vi "set_Al_PID_01.vi"(0 "target flow (sccm)":dbl=76.0 format="%.2f", 1 "Run":bool, 2 "Bubbler In":bool, 3 "Active":bool=TRUE) -> ()   [LabVIEW 2011]
uses:
  <vilib>/Analysis/NI_AALPro.lvlib
panel:
  in  "dtDelay(s)":dbl=161845.394
  out "tTune(s)":dbl=161845.394
  out "Remote":bool
  out "prev dR":dbl
  out "dR":dbl
  out "Polynomial Coefficients":dbl[](array[numeric])=[-1.4185856873488687, 0.3207828308209371, 0.13144453708617976]
  out "Best Polynomial Fit":dbl[](array[numeric])=[-1.4185856873488687, -1.6139263817489564, -1.4535753275096295, -0.934721257482187, -0.06084472416107456, 1.168009538292087, 2.7539547788012695, 4.6979090060566655, 6.9965349595828625, 9.65378216839643, 12.656869913925354, 16.032582856357365, 19.766321537116767, 23.839791139200322, 28.29201256813708, 33.090057519195085, 38.231169600301214, 43.741895001434145, 49.604230522561835, 55.817258155180305, 63.621549699110574, 70.69684374251437, 78.07805746158404, 85.78401348130417, 93.89514333055536, 102.37353612475415, 111.1585051750553, 120.33168859799997, 129.86351160527155, 139.71949074374146, 149.9584374415381, 160.56464392932688, 171.50086747103902, 182.82343196442633, 194.50463604214053, 206.47125485701025, 218.94296295023602, 231.70008578092185, 244.74755627283324, 258.3136303817438]
  out "tFit_array":dbl[](array[numeric])=[-2.0, 0.0]
  out "RFit_array":dbl[](array[numeric])=[73.96843433835814, 74.61000000000001]
  out "error array":dbl[](array[numeric])=[-1.3899999999999864, -1.7800000000000011, -1.3500000000000085, -0.6200000000000045, 0.5699999999999932, 1.6099999999999994, 1.1999999999999886, 0.3199999999999932, -0.13000000000000966, -1.3700000000000045, -1.9499999999999886, -1.7399999999999949, -1.1200000000000045, -0.11999999999999034, 1.759999999999991, 2.3500000000000085, 2.1700000000000017, 1.4099999999999966, 0.4299999999999926, -0.6500000000000057, 54.959999999999994, 55.099999999999994, 55.66000000000001, 56.55000000000001, 57.02000000000001, 58.03, 58.129999999999995, 57.11999999999999, 56.599999999999994, 55.47, 54.80000000000001, 54.84, 55.129999999999995, 55.58, 57.16000000000001, 58.11, 58.09, 57.510000000000005, 56.74000000000001, 55.709999999999994]
  out "dt array":dbl[](array[numeric])=[0.0, -1.1669999999867287, -2.3260000000009313, -3.4940000000060536, -4.657999999995809, -5.820999999996275, -6.98499999998603, -8.14999999999418, -9.314000000013039, -10.478999999992084, -11.64000000001397, -12.807000000000698, -13.973999999987427, -15.135999999998603, -16.304000000003725, -17.469000000011874, -18.630999999993946, -19.796000000002095, -20.95999999999185, -22.122999999992317, -23.497999999992317, -24.67499999998836, -25.84299999999348, -27.005999999993946, -28.176000000006752, -29.347000000008848, -30.510999999998603, -31.679000000003725, -32.84700000000885, -34.0109999999986, -35.178000000014435, -36.345999999990454, -37.5109999999986, -38.679000000003725, -39.84700000000885, -41.00800000000163, -42.18299999998999, -43.35099999999511, -44.513000000006286, -45.68900000001304]
  out "Rtarget array":dbl[](array[numeric])=[76.0, 76.0, 76.0, 76.0, 76.0, 76.0, 76.0, 76.0, 76.0, 76.0, 76.0, 76.0, 76.0, 76.0, 76.0, 76.0, 76.0, 76.0, 76.0, 76.0, 20.0, 20.0, 20.0, 20.0, 20.0, 20.0, 20.0, 20.0, 20.0, 20.0, 20.0, 20.0, 20.0, 20.0, 20.0, 20.0, 20.0, 20.0, 20.0, 20.0]
  out "t array":dbl[](array[numeric])=[161845.394, 161844.227, 161843.068, 161841.9, 161840.736, 161839.573, 161838.409, 161837.244, 161836.08, 161834.915, 161833.754, 161832.587, 161831.42, 161830.258, 161829.09, 161827.925, 161826.763, 161825.598, 161824.434, 161823.271, 161821.896, 161820.719, 161819.551, 161818.388, 161817.218, 161816.047, 161814.883, 161813.715, 161812.547, 161811.383, 161810.216, 161809.048, 161807.883, 161806.715, 161805.547, 161804.386, 161803.211, 161802.043, 161800.881, 161799.705]
  out "R array":dbl[](array[numeric])=[74.61000000000001, 74.22, 74.64999999999999, 75.38, 76.57, 77.61, 77.19999999999999, 76.32, 75.86999999999999, 74.63, 74.05000000000001, 74.26, 74.88, 75.88000000000001, 77.75999999999999, 78.35000000000001, 78.17, 77.41, 76.42999999999999, 75.35, 74.96, 75.1, 75.66000000000001, 76.55000000000001, 77.02000000000001, 78.03, 78.13, 77.11999999999999, 76.6, 75.47, 74.80000000000001, 74.84, 75.13, 75.58, 77.16000000000001, 78.11, 78.09, 77.51, 76.74000000000001, 75.71]
  out "tuning":bool
  in  "Tune":bool
  in  "stop":bool
  in  "Ks":dbl
  out "dt(s)":dbl=1.1669999999867287
  out "windup error":dbl
  out "tPrev":dbl=161845.394
  out "target value":dbl=8.607079070006002
  out "error":dbl=-1.3899999999999864
  out "tNow(s)":dbl=161845.394
  out "weight array":dbl[](array[numeric])=[1.0, 0.3112994401423479, 0.09768570948263659, 0.03037911236430853, 0.009485414272106564, 0.0029646390229553033, 0.0009256632966347818, 0.00028873535962988374, 9.01532101455707e-05, 2.8120829299984297e-05, 8.806680295207305e-06, 2.741514645410681e-06, 8.534319742583924e-07, 2.6700458671159456e-07, 8.303530152421186e-08, 2.5900592293904588e-08, 8.103255033572197e-09, 2.5275888811806865e-09, 7.892010589399871e-10, 2.4666252724157755e-10, 6.236605368793774e-11, 1.9221339918994332e-11, 5.977611753902341e-12, 1.8682854076081917e-12, 5.79854027362869e-13, 1.7978764328562998e-13, 5.613594818436806e-14, 1.74576228867237e-14, 5.429116398891195e-15, 1.6951587510987664e-15, 5.277019701540894e-16, 1.6410913665416056e-16, 5.1189358768628024e-17, 1.5919291471855112e-17, 4.95071333304516e-18, 1.5504290109481995e-18, 4.788019052453027e-19, 1.4890178877471836e-19, 4.6585389077974155e-20, 1.437207306183795e-20]
  in  "# of points to watch":i32=60
  in  "tSmooth(s)":dbl=1.0
  out "first":bool
  out "XY Graph":cluster{"Value":dbl[], "Value":dbl[]}[](graph)=[{"Value"=[0.0, -1.1669999999867287, -2.3260000000009313, -3.4940000000060536, -4.657999999995809, -5.820999999996275, -6.98499999998603, -8.14999999999418, -9.314000000013039, -10.478999999992084, -11.64000000001397, -12.807000000000698, -13.973999999987427, -15.135999999998603, -16.304000000003725, -17.469000000011874, -18.630999999993946, -19.796000000002095, -20.95999999999185, -22.122999999992317, -23.497999999992317, -24.67499999998836, -25.84299999999348, -27.005999999993946, -28.176000000006752, -29.347000000008848, -30.510999999998603, -31.679000000003725, -32.84700000000885, -34.0109999999986, -35.178000000014435, -36.345999999990454, -37.5109999999986, -38.679000000003725, -39.84700000000885, -41.00800000000163, -42.18299999998999, -43.35099999999511, -44.513000000006286, -45.68900000001304], "Value"=[74.61000000000001, 74.22, 74.64999999999999, 75.38, 76.57, 77.61, 77.19999999999999, 76.32, 75.86999999999999, 74.63, 74.05000000000001, 74.26, 74.88, 75.88000000000001, 77.75999999999999, 78.35000000000001, 78.17, 77.41, 76.42999999999999, 75.35, 74.96, 75.1, 75.66000000000001, 76.55000000000001, 77.02000000000001, 78.03, 78.13, 77.11999999999999, 76.6, 75.47, 74.80000000000001, 74.84, 75.13, 75.58, 77.16000000000001, 78.11, 78.09, 77.51, 76.74000000000001, 75.71]}, {"Value"=[-2.0, 0.0], "Value"=[73.96843433835814, 74.61000000000001]}, {"Value"=[0.0, -1.1669999999867287, -2.3260000000009313, -3.4940000000060536, -4.657999999995809, -5.820999999996275, -6.98499999998603, -8.14999999999418, -9.314000000013039, -10.478999999992084, -11.64000000001397, -12.807000000000698, -13.973999999987427, -15.135999999998603, -16.304000000003725, -17.469000000011874, -18.630999999993946, -19.796000000002095, -20.95999999999185, -22.122999999992317, -23.497999999992317, -24.67499999998836, -25.84299999999348, -27.005999999993946, -28.176000000006752, -29.347000000008848, -30.510999999998603, -31.679000000003725, -32.84700000000885, -34.0109999999986, -35.178000000014435, -36.345999999990454, -37.5109999999986, -38.679000000003725, -39.84700000000885, -41.00800000000163, -42.18299999998999, -43.35099999999511, -44.513000000006286, -45.68900000001304], "Value"=[76.0, 76.0, 76.0, 76.0, 76.0, 76.0, 76.0, 76.0, 76.0, 76.0, 76.0, 76.0, 76.0, 76.0, 76.0, 76.0, 76.0, 76.0, 76.0, 76.0, 20.0, 20.0, 20.0, 20.0, 20.0, 20.0, 20.0, 20.0, 20.0, 20.0, 20.0, 20.0, 20.0, 20.0, 20.0, 20.0, 20.0, 20.0, 20.0, 20.0]}]
  out "current value":dbl=8.607079070006002
  in  "Period (s)":dbl=0.5
  out "dValue":dbl=2.1714937580001004
  out "derivative":dbl=0.3207828308209371
  out "integral":dbl=21701.037580001004
  in  "Kd":dbl
  in  "Ki":dbl=0.0001
  in  "Kp":dbl=0.001
  out "actual flow (sccm)":dbl=74.61000000000001 format="%.2f"
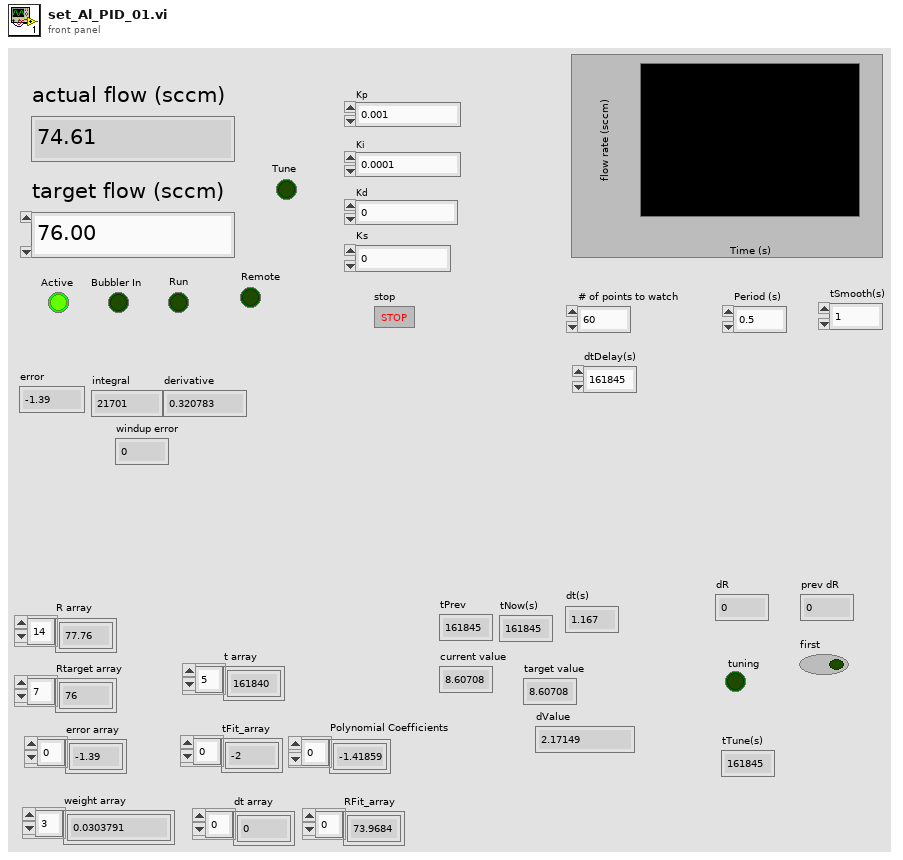
[diagram p1: front panel]
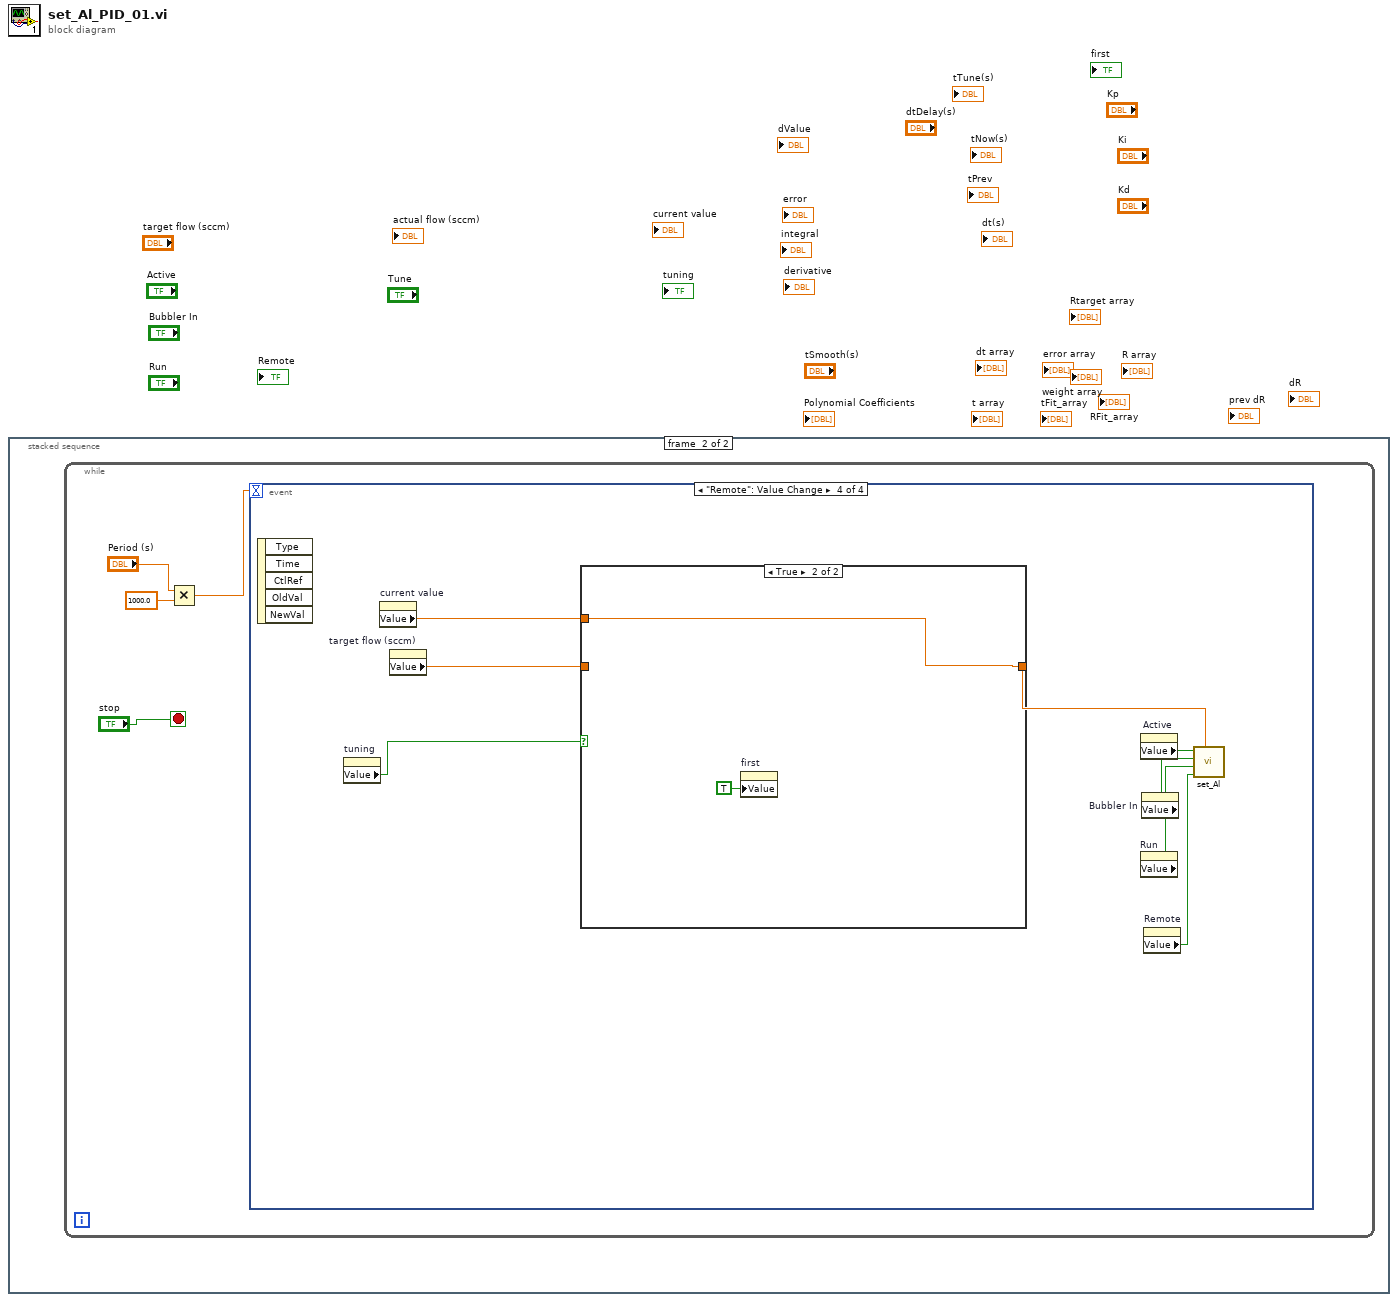
[diagram p0: block diagram]
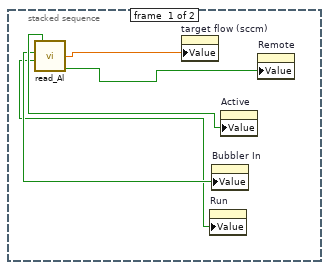
[diagram p2: hidden frame]
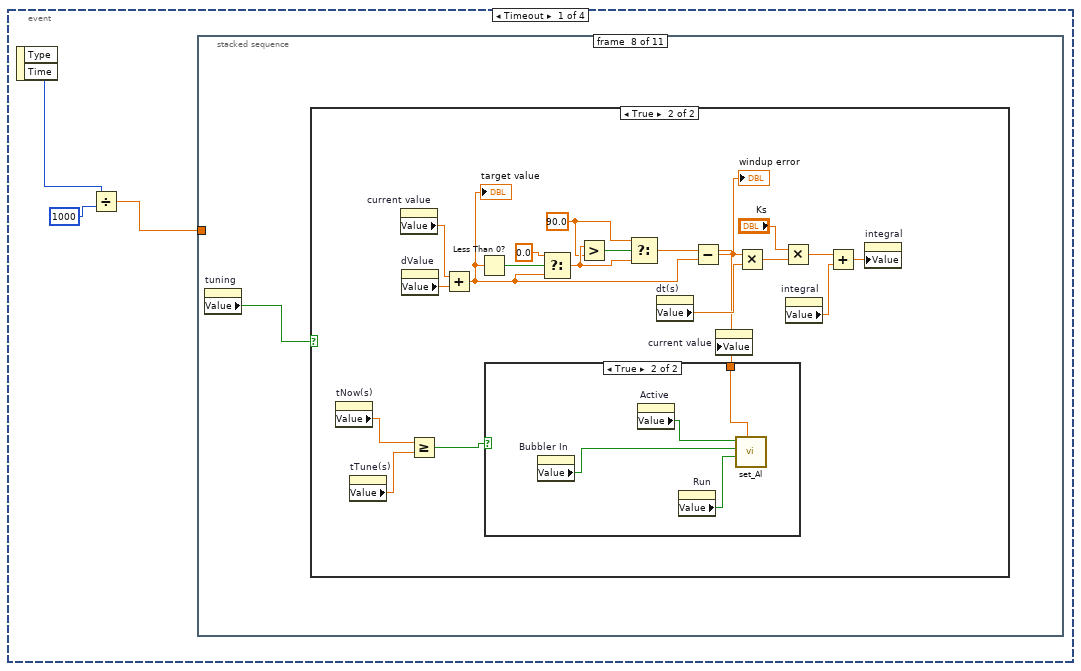
[diagram p3: hidden frame]
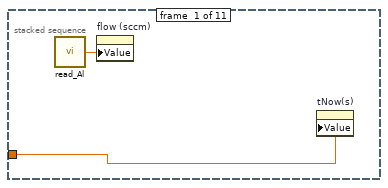
[diagram p4: hidden frame]
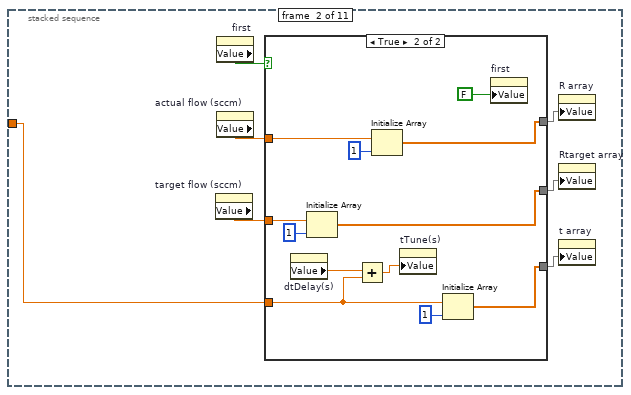
[diagram p5: hidden frame]
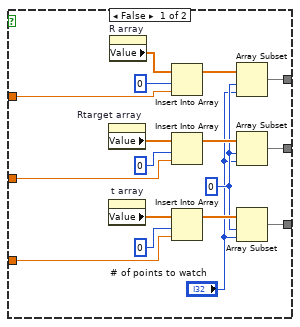
[diagram p6: hidden frame]
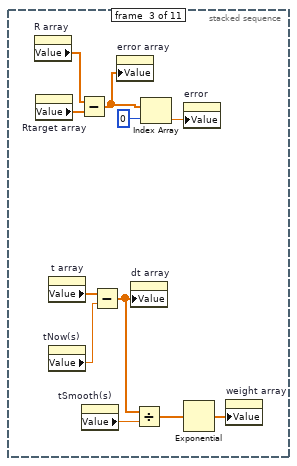
[diagram p7: hidden frame]
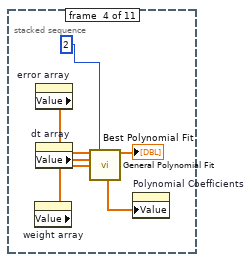
[diagram p8: hidden frame]
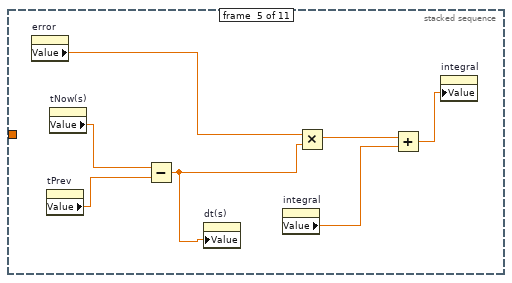
[diagram p9: hidden frame]
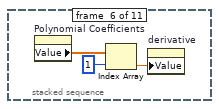
[diagram p10: hidden frame]
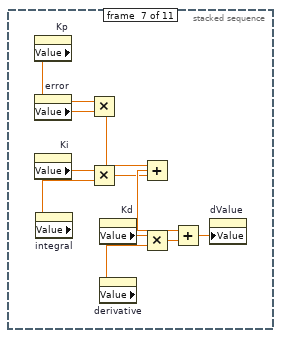
[diagram p11: hidden frame]
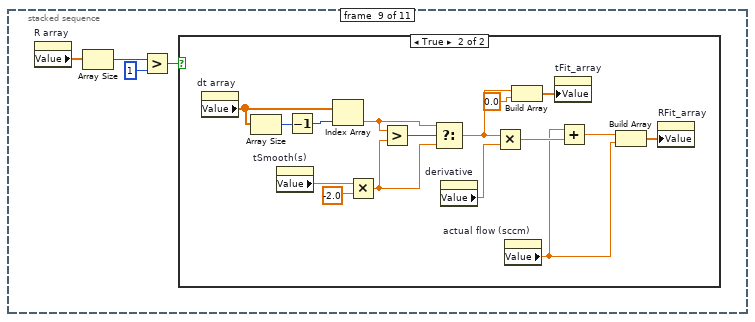
[diagram p14: hidden frame]
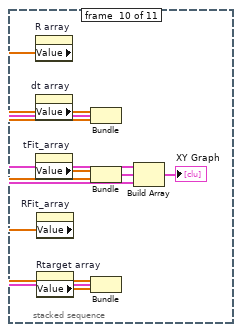
[diagram p16: hidden frame]
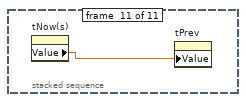
[diagram p17: hidden frame]
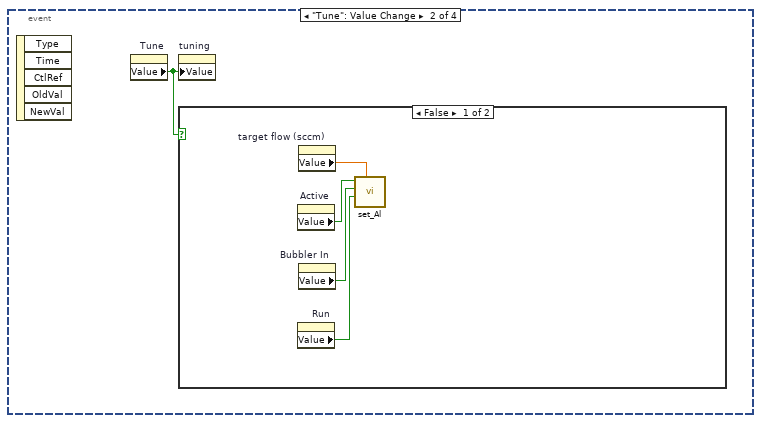
[diagram p18: hidden frame]
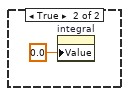
[diagram p19: hidden frame]
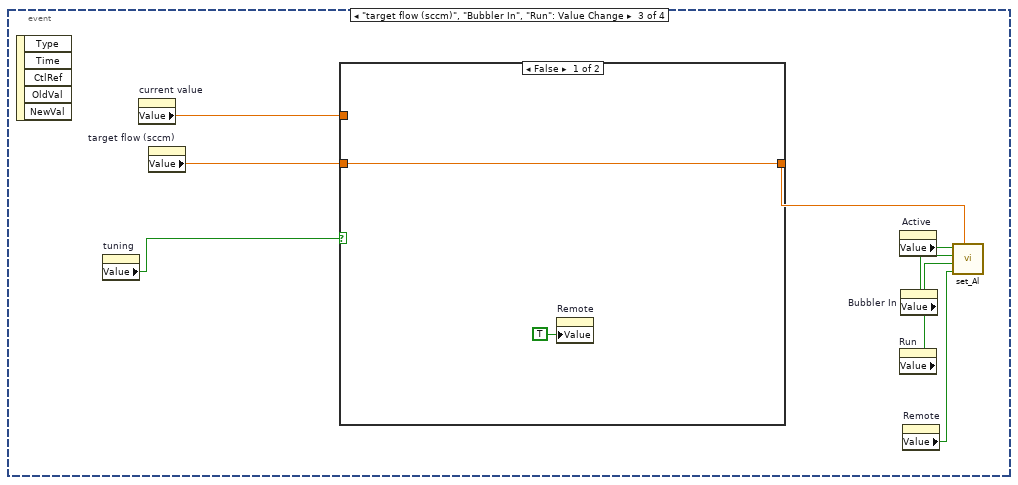
[diagram p20: hidden frame]
diagram:
  n1 = stacked-sequence {
    frame #0 {
      n2 = call "read_Al.vi"() -> ("ALMFC1"=w5:dbl, "Remote"=w1:bool, "Run"=w2:bool, "Bubbler In"=w3:bool, "Active"=w4:bool)
      n3 = property on="target flow (sccm)" class="DigNum (strict)"("Value"=w5) -> ()  [unwired: 2 in, 2 out]
      n4 = property on="Run" class="Bool (strict)"("Value"=w2) -> ()  [unwired: 2 in, 2 out]
      n5 = property on="Bubbler In" class="Bool (strict)"("Value"=w3) -> ()  [unwired: 2 in, 2 out]
      n6 = property on="Active" class="Bool (strict)"("Value"=w4) -> ()  [unwired: 2 in, 2 out]
      n7 = property on="Remote" class="Bool (strict)"("Value"=w1) -> ()  [unwired: 2 in, 2 out]
    }
    frame #1 {
      n8 = while {
        stop <- "stop" stop-if-true
        n9 = Multiply(x="Period (s)", y=1000.0) -> (x*y=w7:dbl)
        n10 = event shown="[3] \"Remote\": Value Change" {
          selector: _ -> [_ _ _ _]
          dyn-events: _ -> [_ _ _ _]
          timeout: w7 -> [_ _ _ _]
          event Timeout {
            n11 = event-data() -> ("Time"=w12:u32)  [unwired: 1 in, 1 out]
            n12 = Divide(x=w12, y=u32 1000) -> (x/y=w10:dbl)
            n13 = stacked-sequence {
              tunnel: w10 -> [w14 w21 _ _ _ _ _ _ _ _ _]
              frame #0 {
                n14 = call "read_Al.vi"() -> ("ALMFC1"=w13:dbl)  [unwired: 4 out]
                n15 = property on="flow (sccm)" class="DigNum (strict)"("Value"=w13) -> ()  [unwired: 2 in, 2 out]
                n16 = property on="tNow(s)" class="DigNum (strict)"("Value"=w14) -> ()  [unwired: 2 in, 2 out]
              }
              frame #1 {
                n17 = property on="target flow (sccm)" class="DigNum (strict)"() -> ("Value"=w16:dbl)  [unwired: 2 in, 2 out]
                n18 = property on="first" class="Bool (strict)"() -> ("Value"=w20:bool)  [unwired: 2 in, 2 out]
                n19 = property on="actual flow (sccm)" class="DigNum (strict)"() -> ("Value"=w19:dbl)  [unwired: 2 in, 2 out]
                n20 = case shown="True" w20 {
                  tunnel: w19 -> [w37 w49]
                  tunnel: [w28 w47] -> w18
                  tunnel: w21 -> [w34 w39]
                  tunnel: [w26 w45] -> w17
                  tunnel: w16 -> [w30 w43]
                  tunnel: [w24 w42] -> w15
                  frame False {
                    w23 = 0 ("index")
                    n21 = property on="Rtarget array" class="Arr (strict)"() -> ("Value"=w31:dbl[])  [unwired: 2 in, 2 out]
                    n22 = property on="t array" class="Arr (strict)"() -> ("Value"=w33:dbl[])  [unwired: 2 in, 2 out]
                    n23 = property on="R array" class="Arr (strict)"() -> ("Value"=w36:dbl[])  [unwired: 2 in, 2 out]
                    n24 = Insert Into Array(array=w36, index=0, new element=w37) -> (w29:dbl[])
                    n25 = Insert Into Array(array=w31, index=0, new element=w30) -> (w25:dbl[])
                    n26 = Insert Into Array(array=w33, index=0, new element=w34) -> (w27:dbl[])
                    n27 = Array Subset(array=w29, index=w23, length="# of points to watch") -> (w28:dbl[])
                    n28 = Array Subset(array=w25, index=w23, length="# of points to watch") -> (w24:dbl[])
                    n29 = Array Subset(array=w27, index=w23, length="# of points to watch") -> (w26:dbl[])
                  }
                  frame True {
                    n30 = property on="dtDelay(s)" class="DigNum (strict)"() -> ("Value"=w40:dbl)  [unwired: 2 in, 2 out]
                    n31 = Initialize Array(w43, 1 ("dimension size")) -> (w42:dbl[])
                    n32 = Add(x=w40, y=w39) -> (x+y=w41:dbl)
                    n33 = Initialize Array(w49, 1 ("dimension size")) -> (w47:dbl[])
                    n34 = property on="tTune(s)" class="DigNum (strict)"("Value"=w41) -> ()  [unwired: 2 in, 2 out]
                    n35 = Initialize Array(w39, 1 ("dimension size")) -> (w45:dbl[])
                    n36 = property on="first" class="Bool (strict)"("Value"=FALSE ("first")) -> ()  [unwired: 2 in, 2 out]
                  }
                }
                n37 = property on="R array" class="Arr (strict)"("Value"=w18) -> ()  [unwired: 2 in, 2 out]
                n38 = property on="Rtarget array" class="Arr (strict)"("Value"=w15) -> ()  [unwired: 2 in, 2 out]
                n39 = property on="t array" class="Arr (strict)"("Value"=w17) -> ()  [unwired: 2 in, 2 out]
              }
              frame #2 {
                n40 = property on="R array" class="Arr (strict)"() -> ("Value"=w55:dbl[])  [unwired: 2 in, 2 out]
                n41 = property on="Rtarget array" class="Arr (strict)"() -> ("Value"=w54:dbl[])  [unwired: 2 in, 2 out]
                n42 = property on="t array" class="Arr (strict)"() -> ("Value"=w61:dbl[])  [unwired: 2 in, 2 out]
                n43 = property on="tNow(s)" class="DigNum (strict)"() -> ("Value"=w60:dbl)  [unwired: 2 in, 2 out]
                n44 = Subtract(x=w55, y=w54) -> (x-y=w53:dbl[])
                n45 = property on="tSmooth(s)" class="DigNum (strict)"() -> ("Value"=w59:dbl)  [unwired: 2 in, 2 out]
                n46 = Subtract(x=w61, y=w60) -> (x-y=w57:dbl[])
                n47 = property on="error array" class="Arr (strict)"("Value"=w53) -> ()  [unwired: 2 in, 2 out]
                n48 = property on="dt array" class="Arr (strict)"("Value"=w57) -> ()  [unwired: 2 in, 2 out]
                n49 = Divide(x=w57, y=w59) -> (x/y=w58:dbl[])
                n50 = Index Array(array=w53, index=0) -> (element=w51:dbl)
                n51 = property on="error" class="DigNum (strict)"("Value"=w51) -> ()  [unwired: 2 in, 2 out]
                n52 = Exponential(1:w58) -> (0:w56:dbl[])
                n53 = property on="weight array" class="Arr (strict)"("Value"=w56) -> ()  [unwired: 2 in, 2 out]
              }
              frame #3 {
                n54 = property on="weight array" class="Arr (strict)"() -> ("Value"=w65:dbl[])  [unwired: 2 in, 2 out]
                n55 = property on="error array" class="Arr (strict)"() -> ("Value"=w67:dbl[])  [unwired: 2 in, 2 out]
                n56 = property on="dt array" class="Arr (strict)"() -> ("Value"=w66:dbl[])  [unwired: 2 in, 2 out]
                n57 = call <vilib>:"General Polynomial Fit.vi"("Y"=w67, "polynomial order"=2, "X"=w66, "Weight"=w65) -> ("Best Polynomial Fit"=→"Best Polynomial Fit":dbl[], "Polynomial Coefficients"=w62:dbl[])  [unwired: 8 in, 2 out]
                n58 = property on="Polynomial Coefficients" class="Arr (strict)"("Value"=w62) -> ()  [unwired: 2 in, 2 out]
              }
              frame #4 {
                n59 = property on="error" class="DigNum (strict)"() -> ("Value"=w70:dbl)  [unwired: 2 in, 2 out]
                n60 = property on="tPrev" class="DigNum (strict)"() -> ("Value"=w69:dbl)  [unwired: 2 in, 2 out]
                n61 = property on="tNow(s)" class="DigNum (strict)"() -> ("Value"=w68:dbl)  [unwired: 2 in, 2 out]
                n62 = Subtract(x=w68, y=w69) -> (x-y=w74:dbl)
                n63 = property on="dt(s)" class="DigNum (strict)"("Value"=w74) -> ()  [unwired: 2 in, 2 out]
                n64 = property on="integral" class="DigNum (strict)"() -> ("Value"=w72:dbl)  [unwired: 2 in, 2 out]
                n65 = Multiply(x=w70, y=w74) -> (x*y=w71:dbl)
                n66 = Add(x=w71, y=w72) -> (x+y=w73:dbl)
                n67 = property on="integral" class="DigNum (strict)"("Value"=w73) -> ()  [unwired: 2 in, 2 out]
              }
              frame #5 {
                n68 = property on="Polynomial Coefficients" class="Arr (strict)"() -> ("Value"=w77:dbl[])  [unwired: 2 in, 2 out]
                n69 = Index Array(array=w77, index=1) -> (element=w75:dbl)
                n70 = property on="derivative" class="DigNum (strict)"("Value"=w75) -> ()  [unwired: 2 in, 2 out]
              }
              frame #6 {
                n71 = property on="Kp" class="DigNum (strict)"() -> ("Value"=w78:dbl)  [unwired: 2 in, 2 out]
                n72 = property on="error" class="DigNum (strict)"() -> ("Value"=w88:dbl)  [unwired: 2 in, 2 out]
                n73 = property on="Ki" class="DigNum (strict)"() -> ("Value"=w79:dbl)  [unwired: 2 in, 2 out]
                n74 = property on="integral" class="DigNum (strict)"() -> ("Value"=w80:dbl)  [unwired: 2 in, 2 out]
                n75 = Multiply(x=w78, y=w88) -> (x*y=w83:dbl)
                n76 = Multiply(x=w79, y=w80) -> (x*y=w84:dbl)
                n77 = property on="Kd" class="DigNum (strict)"() -> ("Value"=w81:dbl)  [unwired: 2 in, 2 out]
                n78 = property on="derivative" class="DigNum (strict)"() -> ("Value"=w82:dbl)  [unwired: 2 in, 2 out]
                n79 = Add(x=w83, y=w84) -> (x+y=w86:dbl)
                n80 = Multiply(x=w81, y=w82) -> (x*y=w85:dbl)
                n81 = Add(x=w86, y=w85) -> (x+y=w87:dbl)
                n82 = property on="dValue" class="DigNum (strict)"("Value"=w87) -> ()  [unwired: 2 in, 2 out]
              }
              frame #7 {
                n83 = property on="tuning" class="Bool (strict)"() -> ("Value"=w89:bool)  [unwired: 2 in, 2 out]
                n84 = case shown="True" w89 {
                  frame False {
                  }
                  frame True {
                    w102 = 90.0 ("y")
                    n85 = property on="tNow(s)" class="DigNum (strict)"() -> ("Value"=w92:dbl)  [unwired: 2 in, 2 out]
                    n86 = property on="tTune(s)" class="DigNum (strict)"() -> ("Value"=w91:dbl)  [unwired: 2 in, 2 out]
                    n87 = property on="current value" class="DigNum (strict)"() -> ("Value"=w108:dbl)  [unwired: 2 in, 2 out]
                    n88 = property on="dValue" class="DigNum (strict)"() -> ("Value"=w107:dbl)  [unwired: 2 in, 2 out]
                    n89 = Greater Or Equal?(x=w92, y=w91) -> (x >= y?=w90:bool)
                    n90 = Add(x=w108, y=w107) -> (x+y=w94:dbl)
                    "target value" <- w94
                    n91 = Less Than 0?(x=w94) -> (x < 0?=w106:bool)
                    n92 = Select(t=0.0, s=w106, f=w94) -> (s? t:f=w103:dbl)
                    n93 = Greater?(x=w103, y=w102) -> (0:w104:bool)
                    n94 = Select(t=w102, s=w104, f=w103) -> (s? t:f=w93:dbl)
                    n95 = case shown="True" w90 {
                      tunnel: w93 -> [_ w112]
                      frame False {
                      }
                      frame True {
                        n96 = property on="Bubbler In" class="Bool (strict)"() -> ("Value"=w109:bool)  [unwired: 2 in, 2 out]
                        n97 = property on="Active" class="Bool (strict)"() -> ("Value"=w110:bool)  [unwired: 2 in, 2 out]
                        n98 = property on="Run" class="Bool (strict)"() -> ("Value"=w111:bool)  [unwired: 2 in, 2 out]
                        n99 = call "set_Al.vi"("ALMFC1"=w112, "Run"=w111, "Bubbler In"=w109, "Active"=w110) -> ()  [unwired: 6 in]
                      }
                    }
                    n100 = property on="dt(s)" class="DigNum (strict)"() -> ("Value"=w100:dbl)  [unwired: 2 in, 2 out]
                    n101 = Subtract(x=w93, y=w94) -> (x-y=w101:dbl)
                    "windup error" <- w101
                    n102 = property on="current value" class="DigNum (strict)"("Value"=w93) -> ()  [unwired: 2 in, 2 out]
                    n103 = Multiply(x=w101, y=w100) -> (x*y=w99:dbl)
                    n104 = Multiply(x="Ks", y=w99) -> (x*y=w97:dbl)
                    n105 = property on="integral" class="DigNum (strict)"() -> ("Value"=w96:dbl)  [unwired: 2 in, 2 out]
                    n106 = Add(x=w97, y=w96) -> (x+y=w95:dbl)
                    n107 = property on="integral" class="DigNum (strict)"("Value"=w95) -> ()  [unwired: 2 in, 2 out]
                  }
                }
              }
              frame #8 {
                n108 = property on="R array" class="Arr (strict)"() -> ("Value"=w113:dbl[])  [unwired: 2 in, 2 out]
                n109 = Array Size(array=w113) -> (size(s)=w114:i32)
                n110 = Greater?(x=w114, y=1) -> (0:w116:bool)
                n111 = case shown="True" w116 {
                  frame False {
                  }
                  frame True {
                    n112 = property on="dt array" class="Arr (strict)"() -> ("Value"=w124:dbl[])  [unwired: 2 in, 2 out]
                    n113 = Array Size(array=w124) -> (size(s)=w132:i32)
                    n114 = property on="tSmooth(s)" class="DigNum (strict)"() -> ("Value"=w126:dbl)  [unwired: 2 in, 2 out]
                    n115 = Decrement(x=w132) -> (x-1=w131:i32)
                    n116 = Index Array(array=w124, index=w131) -> (element=w125:dbl)
                    n117 = Multiply(x=w126, y=-2.0) -> (x*y=w117:dbl)
                    n118 = Greater?(x=w125, y=w117) -> (0:w128:bool)
                    n119 = Select(t=w125, s=w128, f=w117) -> (s? t:f=w121:dbl)
                    n120 = property on="derivative" class="DigNum (strict)"() -> ("Value"=w130:dbl)  [unwired: 2 in, 2 out]
                    n121 = Multiply(x=w121, y=w130) -> (x*y=w129:dbl)
                    n122 = property on="actual flow (sccm)" class="DigNum (strict)"() -> ("Value"=w123:dbl)  [unwired: 2 in, 2 out]
                    n123 = Build Array(w121, 0.0 ("element")) -> (w119:dbl[])
                    n124 = property on="tFit_array" class="Arr (strict)"("Value"=w119) -> ()  [unwired: 2 in, 2 out]
                    n125 = Add(x=w123, y=w129) -> (x+y=w122:dbl)
                    n126 = Build Array(w122, w123) -> (w118:dbl[])
                    n127 = property on="RFit_array" class="Arr (strict)"("Value"=w118) -> ()  [unwired: 2 in, 2 out]
                  }
                }
              }
              frame #9 {
                n128 = property on="R array" class="Arr (strict)"() -> ("Value"=w141:dbl[])  [unwired: 2 in, 2 out]
                n129 = property on="dt array" class="Arr (strict)"() -> ("Value"=w133:dbl[])  [unwired: 2 in, 2 out]
                n130 = property on="tFit_array" class="Arr (strict)"() -> ("Value"=w140:dbl[])  [unwired: 2 in, 2 out]
                n131 = property on="RFit_array" class="Arr (strict)"() -> ("Value"=w139:dbl[])  [unwired: 2 in, 2 out]
                n132 = property on="Rtarget array" class="Arr (strict)"() -> ("Value"=w135:dbl[])  [unwired: 2 in, 2 out]
                n133 = Bundle("Value"=w133, "Value"=w141) -> (w138:cluster{"Value":dbl[], "Value":dbl[]})  [unwired: 1 in]
                n134 = Bundle("Value"=w140, "Value"=w139) -> (w137:cluster{"Value":dbl[], "Value":dbl[]})  [unwired: 1 in]
                n135 = Bundle("Value"=w133, "Value"=w135) -> (w134:cluster{"Value":dbl[], "Value":dbl[]})  [unwired: 1 in]
                n136 = Build Array(w138, w137, w134) -> (→"XY Graph":cluster{"Value":dbl[], "Value":dbl[]}[])
              }
              frame #10 {
                n137 = property on="tNow(s)" class="DigNum (strict)"() -> ("Value"=w142:dbl)  [unwired: 2 in, 2 out]
                n138 = property on="tPrev" class="DigNum (strict)"("Value"=w142) -> ()  [unwired: 2 in, 2 out]
              }
            }
          }
          event "Tune": Value Change {
            n139 = event-data() -> ()  [unwired: 1 in, 5 out]
            n140 = property on="Tune" class="Bool (strict)"() -> ("Value"=w143:bool)  [unwired: 2 in, 2 out]
            n141 = property on="tuning" class="Bool (strict)"("Value"=w143) -> ()  [unwired: 2 in, 2 out]
            n142 = case shown="False" w143 {
              frame False {
                n143 = property on="Active" class="Bool (strict)"() -> ("Value"=w144:bool)  [unwired: 2 in, 2 out]
                n144 = property on="Run" class="Bool (strict)"() -> ("Value"=w146:bool)  [unwired: 2 in, 2 out]
                n145 = property on="target flow (sccm)" class="DigNum (strict)"() -> ("Value"=w147:dbl)  [unwired: 2 in, 2 out]
                n146 = property on="Bubbler In" class="Bool (strict)"() -> ("Value"=w145:bool)  [unwired: 2 in, 2 out]
                n147 = call "set_Al.vi"("ALMFC1"=w147, "Run"=w146, "Bubbler In"=w145, "Active"=w144) -> ()  [unwired: 6 in]
              }
              frame True {
                n148 = property on="integral" class="DigNum (strict)"("Value"=0.0 ("integral")) -> ()  [unwired: 2 in, 2 out]
              }
            }
          }
          event "target flow (sccm)", "Bubbler In", "Run": Value Change {
            n149 = event-data() -> ()  [unwired: 1 in, 5 out]
            n150 = property on="tuning" class="Bool (strict)"() -> ("Value"=w155:bool)  [unwired: 2 in, 2 out]
            n151 = property on="current value" class="DigNum (strict)"() -> ("Value"=w150:dbl)  [unwired: 2 in, 2 out]
            n152 = property on="target flow (sccm)" class="DigNum (strict)"() -> ("Value"=w156:dbl)  [unwired: 2 in, 2 out]
            n153 = case shown="False" w155 {
              tunnel: w156 -> [w158 _]
              tunnel: [w158 w161] -> w151
              tunnel: w150 -> [_ w161]
              frame False {
                n154 = property on="Remote" class="Bool (strict)"("Value"=TRUE ("Remote")) -> ()  [unwired: 2 in, 2 out]
              }
              frame True {
                n155 = property on="first" class="Bool (strict)"("Value"=TRUE ("first")) -> ()  [unwired: 2 in, 2 out]
                n156 = property on="Remote" class="Bool (strict)"("Value"=TRUE ("Remote")) -> ()  [unwired: 2 in, 2 out]
              }
            }
            n157 = property on="Active" class="Bool (strict)"() -> ("Value"=w152:bool)  [unwired: 2 in, 2 out]
            n158 = property on="Run" class="Bool (strict)"() -> ("Value"=w154:bool)  [unwired: 2 in, 2 out]
            n159 = property on="Bubbler In" class="Bool (strict)"() -> ("Value"=w153:bool)  [unwired: 2 in, 2 out]
            n160 = property on="Remote" class="Bool (strict)"() -> ("Value"=w149:bool)  [unwired: 2 in, 2 out]
            n161 = call "set_Al.vi"("ALMFC1"=w151, "Remote"=w149, "Run"=w154, "Bubbler In"=w153, "Active"=w152) -> ()  [unwired: 5 in]
          }
          event "Remote": Value Change {
            n162 = event-data() -> ()  [unwired: 1 in, 5 out]
            n163 = property on="tuning" class="Bool (strict)"() -> ("Value"=w168:bool)  [unwired: 2 in, 2 out]
            n164 = property on="current value" class="DigNum (strict)"() -> ("Value"=w163:dbl)  [unwired: 2 in, 2 out]
            n165 = property on="target flow (sccm)" class="DigNum (strict)"() -> ("Value"=w169:dbl)  [unwired: 2 in, 2 out]
            n166 = case shown="True" w168 {
              tunnel: w169 -> [w170 _]
              tunnel: [w170 w172] -> w164
              tunnel: w163 -> [_ w172]
              frame False {
              }
              frame True {
                n167 = property on="first" class="Bool (strict)"("Value"=TRUE ("first")) -> ()  [unwired: 2 in, 2 out]
              }
            }
            n168 = property on="Active" class="Bool (strict)"() -> ("Value"=w165:bool)  [unwired: 2 in, 2 out]
            n169 = property on="Run" class="Bool (strict)"() -> ("Value"=w167:bool)  [unwired: 2 in, 2 out]
            n170 = property on="Bubbler In" class="Bool (strict)"() -> ("Value"=w166:bool)  [unwired: 2 in, 2 out]
            n171 = property on="Remote" class="Bool (strict)"() -> ("Value"=w162:bool)  [unwired: 2 in, 2 out]
            n172 = call "set_Al.vi"("ALMFC1"=w164, "Remote"=w162, "Run"=w167, "Bubbler In"=w166, "Active"=w165) -> ()  [unwired: 5 in]
          }
        }
      }
    }
  }
